vi "license agreement.vi"(3 "year":u16) -> (0 "Accepted":bool, 1 "License":string)   [LabVIEW 2015]
panel:
  out "title":string
  in  "OK Button":bool
  in  "I do NOT accept terms of the agreement":bool=TRUE
  in  "I accept terms of the agreement":bool
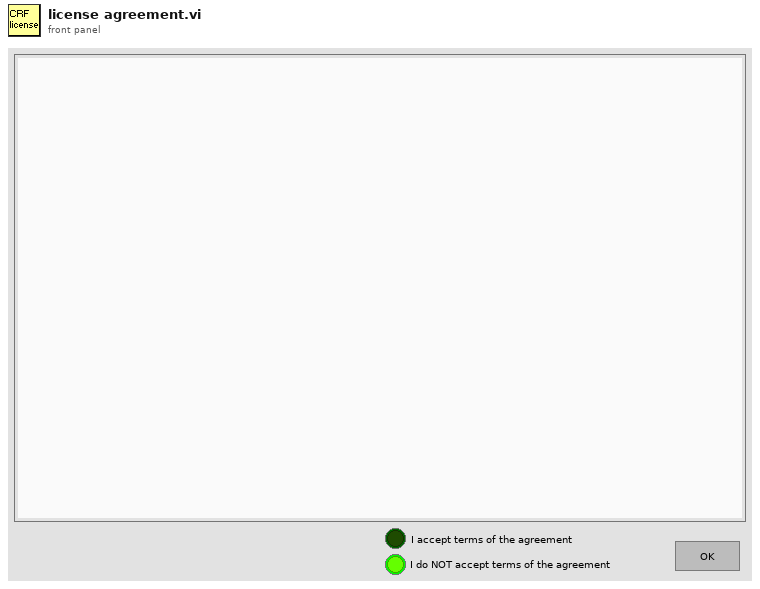
[diagram p1: front panel]
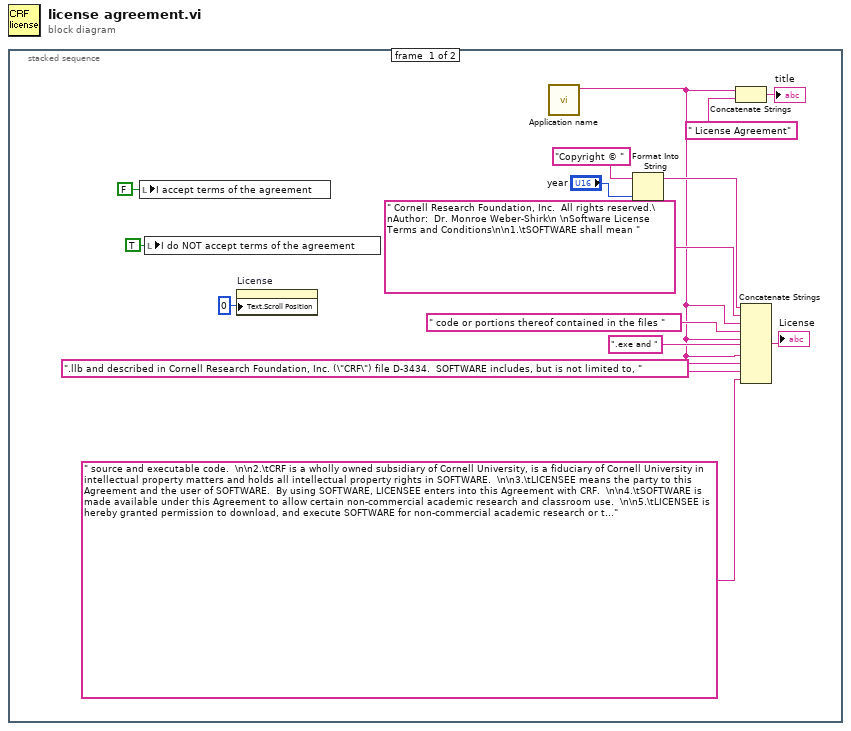
[diagram p0: block diagram]
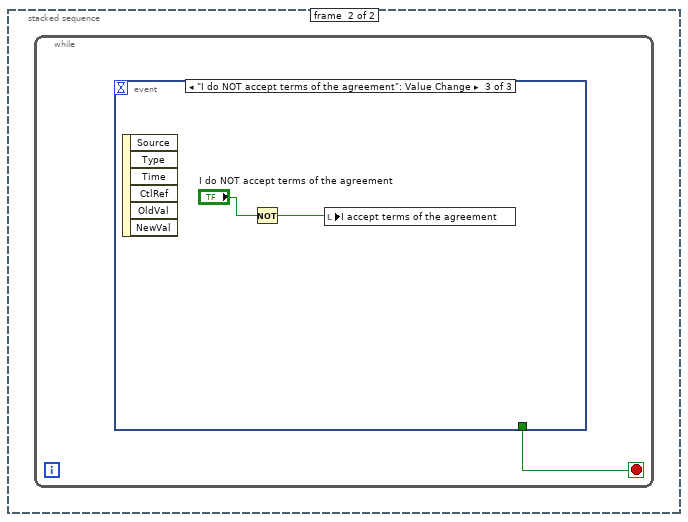
[diagram p2: hidden frame]
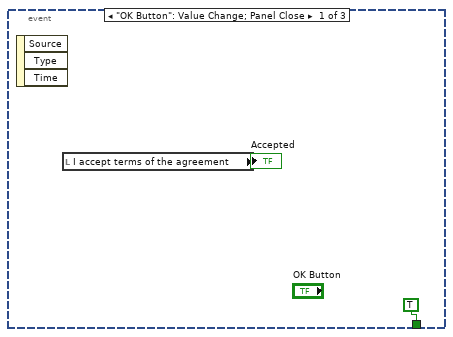
[diagram p3: hidden frame]
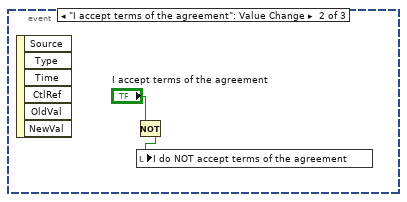
[diagram p4: hidden frame]
diagram:
  n1 = stacked-sequence {
    frame #0 {
      n2 = local write "I accept terms of the agreement"(FALSE ("I accept terms of the agreement")) -> ()
      n3 = local write "I do NOT accept terms of the agreement"(TRUE ("I do NOT accept terms of the agreement")) -> ()
      n4 = property on="License" class="Str"("Text.Scroll Position"=u32 0) -> ()  [unwired: 2 in, 2 out]
      n5 = call "Application name.vi"() -> ("application name"=w1:string)  [unwired: 5 in, 2 out]
      n6 = Format Into String(initial string="Copyright © ", "year") -> (resulting string=w11:string)  [unwired: 2 in, 1 out]
      n7 = Concatenate Strings(w1, " License Agreement" ("string")) -> (→"title":string)
      n8 = Concatenate Strings(w11, " Cornell Research Foundation, Inc.  All rights reserved.\nAuthor:  Dr. Monroe Weber-Shirk\n \nSoftware License Terms and Conditions\n\n1.\tSOFTWARE shall mean ", w1, " code or portions thereof contained in the files ", w1, ".exe and ", w1, ".llb and described in Cornell Research Foundation, Inc. (\"CRF\") file D-3434.  SOFTWARE includes, but is not limited to, ", w1, " source and executable code.  \n\n2.\tCRF is a wholly owned subsidiary of Cornell University, is a fiduciary of Cornell University in intellectual property matters and holds all intellectual property rights in SOFTWARE.  \n\n3.\tLICENSEE means the party to this Agreement and the user of SOFTWARE.  By using SOFTWARE, LICENSEE enters into this Agreement with CRF.  \n\n4.\tSOFTWARE is made available under this Agreement to allow certain non-commercial academic research and classroom use.  \n\n5.\tLICENSEE is hereby granted permission to download, and execute SOFTWARE for non-commercial academic research or teaching purposes provided that this notice accompanies all copies of SOFTWARE.  \n\n6.\tLICENSEE agrees that the export of SOFTWARE from the United States may require approval from the U.S. government and failure to obtain such approval will result in the immediate termination of this license and may result in criminal liability under U.S. laws.\n\n7.\tCRF provides SOFTWARE on an \"as is\" basis.  CRF does not warrant, guarantee, or make any representations regarding the use or results of SOFTWARE with respect to its correctness, accuracy, reliability or performance.  The entire risk of the use and performance of SOFTWARE is assumed by LICENSEE.  ALL WARRANTIES INCLUDING, WITHOUT LIMITATION, ANY WARRANTY OF FITNESS FOR A PARTICULAR PURPOSE OR MERCHANTABILITY AND ANY WARRANTY OF NONINFRINGEMENT OF PATENTS, COPYRIGHTS, OR ANY OTHER INTELLECTUAL PROPERTY RIGHT ARE HEREBY EXCLUDED.\n\n8.\tLICENSEE understands and agrees that neither CRF nor Cornell University is under any obligation to provide maintenance, support or update services, notices of latent defects, correction of defects, or future versions for SOFTWARE.  \n\n9.\tEven if advised of the possibility of damages, under no circumstances shall CRF or Cornell University individually or jointly be liable to LICENSEE or any third party for damages of any character, including, without limitation, direct, indirect, incidental, consequential or special damages, loss of profits, loss of use, loss of goodwill, computer failure or malfunction.  LICENSEE agrees to indemnify and hold harmless CRF and Cornell University for any and all liability CRF or Cornell University may incur as a result of use of SOFTWARE by LICENSEE. ") -> (→"License":string)
    }
    frame #1 {
      n9 = while {
        stop <- w16 stop-if-true
        n10 = event shown="[2] \"I do NOT accept terms of the agreement\": Value Change" {
          selector: _ -> [_ _ _]
          dyn-events: _ -> [_ _ _]
          timeout: _ -> [_ _ _]
          tunnel: [TRUE ("OK Button") _ _] -> w16
          event "OK Button": Value Change; Panel Close {
            n11 = event-data() -> ()  [unwired: 1 in, 3 out]
            n12 = local read "I accept terms of the agreement"() -> (→"Accepted":bool)
          }
          event "I accept terms of the agreement": Value Change {
            n13 = event-data() -> ()  [unwired: 1 in, 6 out]
            n14 = Not(x="I accept terms of the agreement") -> (.not. x?=w19:bool)
            n15 = local write "I do NOT accept terms of the agreement"(w19) -> ()
          }
          event "I do NOT accept terms of the agreement": Value Change {
            n16 = event-data() -> ()  [unwired: 1 in, 6 out]
            n17 = Not(x="I do NOT accept terms of the agreement") -> (.not. x?=w21:bool)
            n18 = local write "I accept terms of the agreement"(w21) -> ()
          }
        }
      }
    }
  }
